vi "UpdateHud.vi"(8 "error in (no error)":errorcluster, 9 "Ticks Elapsed (ms)":u32, 10 "Pitch Delta":sgl, 11 "Player in":refnum<class "Player.lvclass">) -> (0 "error out":errorcluster, 3 "Player out":refnum<class "Player.lvclass">)   [LabVIEW 2015, in "Player.lvclass"]
uses:
  Player.lvclass
  Player.lvclass/Player.ctl
  3D Object/3D Object.lvclass
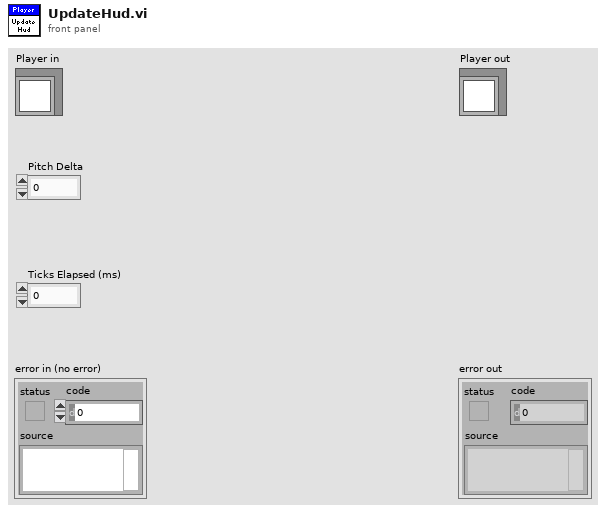
[diagram p1: front panel]
types:
  T1 = typedef "LVSceneTextAlignment.ctl" = cluster{"Horizontal Alignment":enum8{"Left", "Right", "Center"}, "Vertical Alignment":enum8{"Top", "Bottom", "Center", "Base Line", "Bottom Base Line"}}
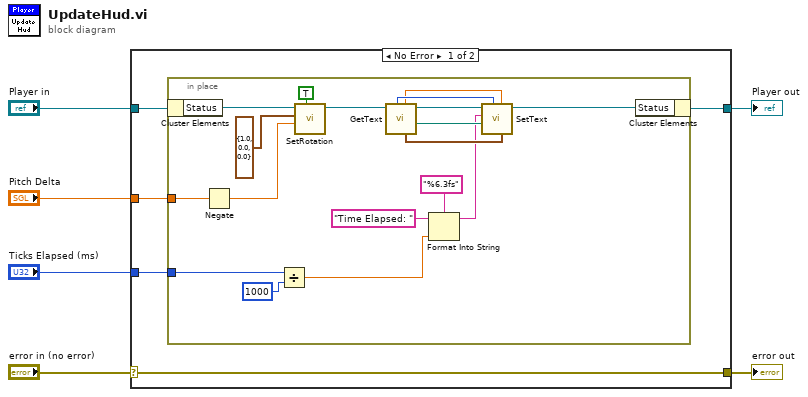
[diagram p0: block diagram]
diagram:
  n1 = case shown="No Error" "error in (no error)" {
    selector: "error in (no error)" -> [w8 w31]
    tunnel: [w8 w31] -> w5
    tunnel: [w10 w30] -> w3
    tunnel: "Player in" -> [w11 w30]
    tunnel: "Pitch Delta" -> [w9 _]
    tunnel: "Ticks Elapsed (ms)" -> [w7 _]
    frame No Error {
      n2 = in-place {
        in-place-border: w9 -> [w29]
        in-place-border: w7 -> [w14]
        n3 = in-place-cluster #1(w11) -> ("Status"=w25:refnum<class "3D Object.lvclass">)
        n4 = Negate(x=w29) -> (-x=w28:sgl)
        n5 = Divide(x=w14, y=u32 1000) -> (x/y=w12:dbl)
        n6 = call "SetRotation.vi"("Relative?"=TRUE, "Angle"=w28, "Axis"=cluster{"X":sgl, "Y":sgl, "Z":sgl} {"X"=1.0, "Y"=0.0, "Z"=0.0}, "3D Object in"=w25) -> ("3D Object out"=w23:refnum<class "3D Object.lvclass">)  [unwired: 6 in, 1 out]
        n7 = call "GetText.vi"("3D Object in"=w23) -> ("Font Path"=w21:path, "3D Object out"=w22:refnum<class "3D Object.lvclass">, "Alignment"=w20:T1, "Alpha"=w18:sgl, "Color"=w19:u32)  [unwired: 4 in, 2 out]
        n8 = Format Into String(format string="%6.3fs", initial string="Time Elapsed: " ("Text"), w12) -> (resulting string=w15:string)  [unwired: 1 in, 1 out]
        n9 = call "SetText.vi"("Alignment"=w20, "Alpha"=w18, "Color"=w19, "Font Path"=w21, "Text"=w15, "3D Object in"=w22) -> ("3D Object out"=w24:refnum<class "3D Object.lvclass">)  [unwired: 4 in, 1 out]
        n10 = in-place-cluster #1("Status"=w24) -> (w10:refnum<class "Player.lvclass">)
      }
    }
    frame Error {
    }
  }
  "error out" <- w5
  "Player out" <- w3
